vi "DivisionUI.vi"(0 "Divide in":refnum<class "Divide.lvclass">, 1 "B":dbl, 5 "A":dbl, 7 "user event out":refnum<user-event>, 9 "event source":refnum<user-event>, 11 "error in (no error)":errorcluster, 12 "Calculate":bool) -> (4 "Divide out":refnum<class "Divide.lvclass">, 6 "C":dbl, 15 "error out":errorcluster)   [LabVIEW 2023, in "Divide.lvclass"]
uses:
  Divide.lvclass
  C:/Users/santharu.subramanian/Documents/LV New Assignments/DVR in OOPS/Classes/Arithmetic/Arithmetic.lvclass
  Arithmetic/Arithmetic.lvclass
  Divide.lvclass/Divide.ctl
panel:
  # "DIVISION"
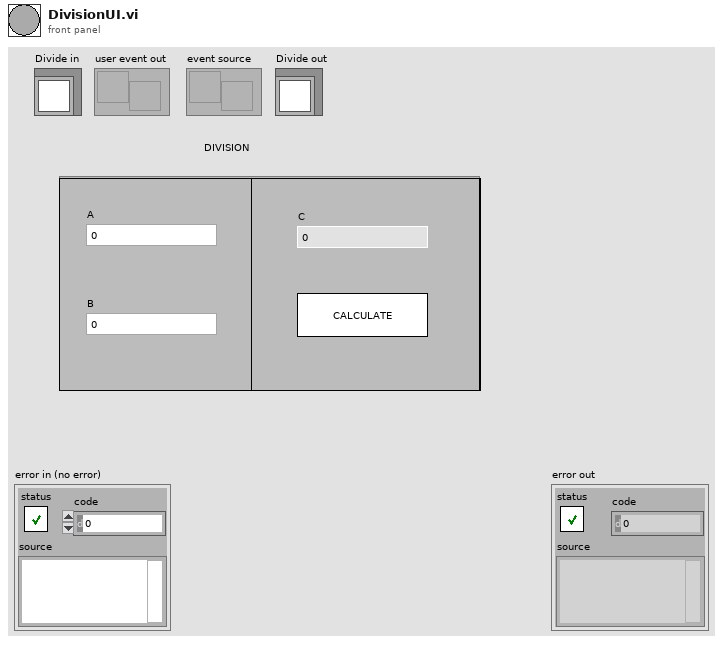
[diagram p1: front panel]
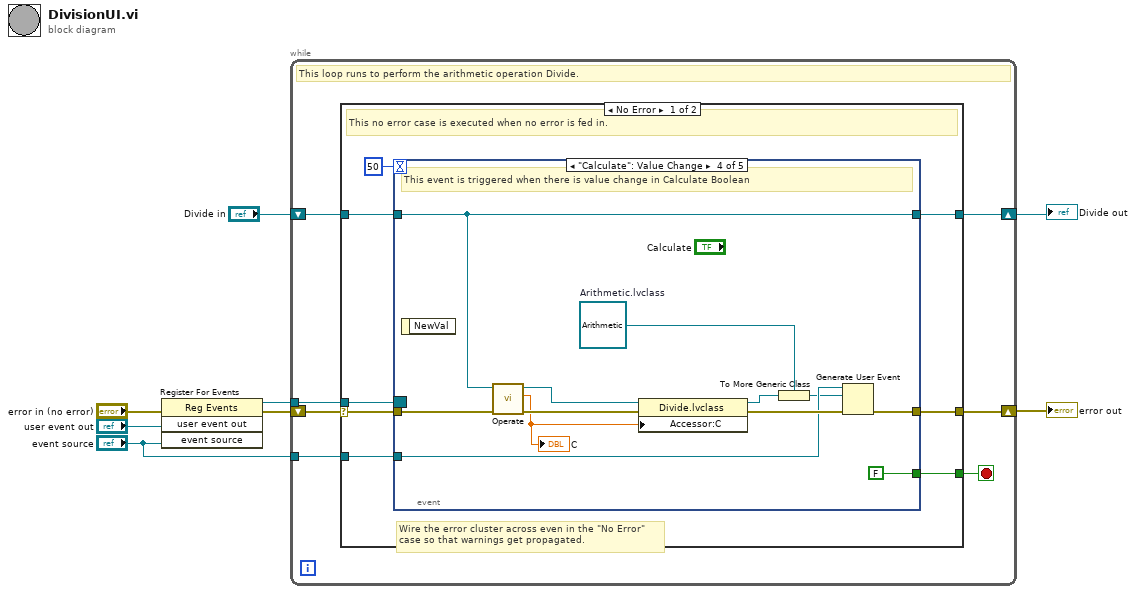
[diagram p0: block diagram]
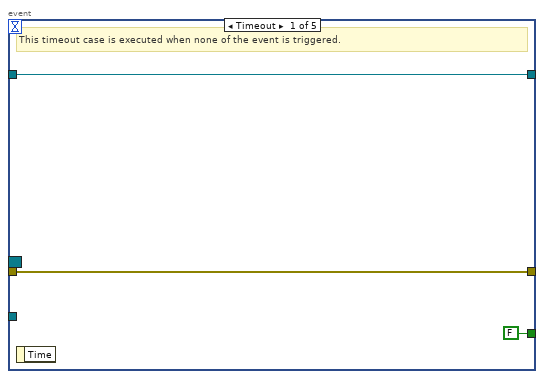
[diagram p2: hidden frame]
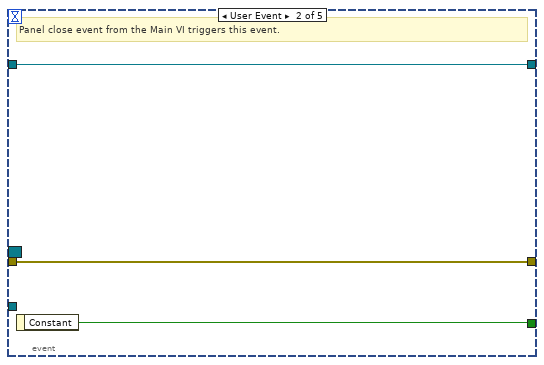
[diagram p3: hidden frame]
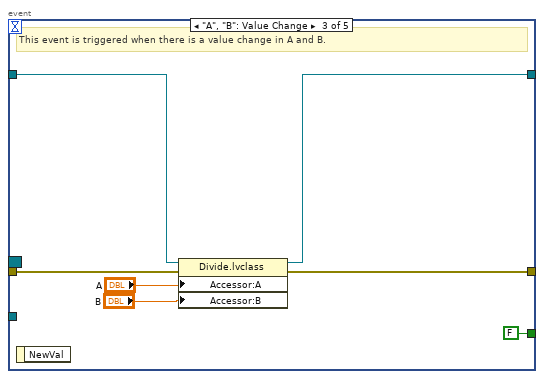
[diagram p4: hidden frame]
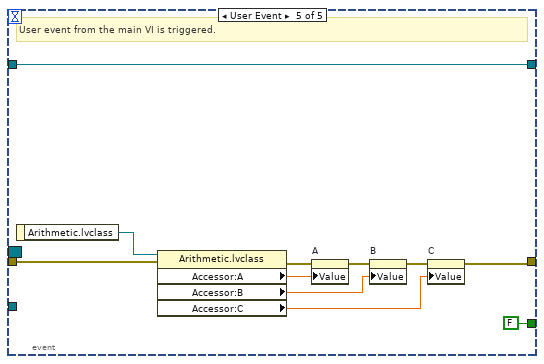
[diagram p5: hidden frame]
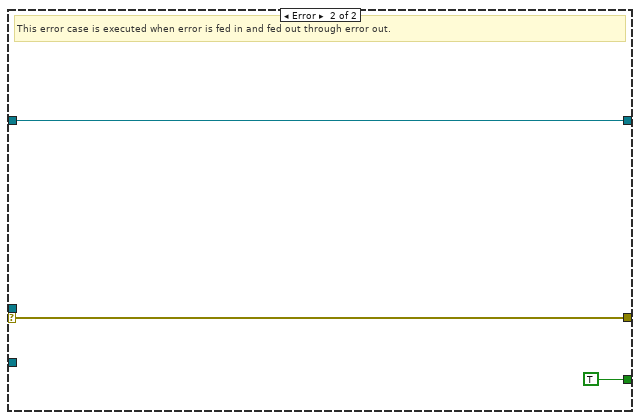
[diagram p6: hidden frame]
diagram:
  # "Wire the error cluster across even in the \"No Error\"\ncase so that warnings get propagated."
  n1 = register-events(error in="error in (no error)", "user event out", "event source") -> (reference out=w3:refnum<event-registration>, error out=w4:errorcluster)  [unwired: 1 in]
  n2 = while {
    shift-right: [w14] -> w6
    shift-left: w4 -> [w15]
    shift-right: [w12] -> w7
    shift-left: "Divide in" -> [w13]
    tunnel: w3 -> [w11]
    tunnel: "event source" -> [w9]
    stop <- w10 stop-if-true
    # "This loop runs to perform the arithmetic operation Divide."
    n3 = case shown="No Error" w15 {
      selector: w15 -> [w23 w62]
      tunnel: [w22 w62] -> w14
      tunnel: [w20 w61] -> w12
      tunnel: w13 -> [w21 w61]
      tunnel: w11 -> [w18 _]
      tunnel: [w17 TRUE] -> w10
      tunnel: w9 -> [w16 _]
      frame No Error {
        # "This no error case is executed when no error is fed in."
        n4 = event shown="[3] \"Calculate\": Value Change" {
          selector: w18 -> [_ _ _ _ _]
          dyn-events: _ -> [_ _ _ _ _]
          timeout: 50 -> [_ _ _ _ _]
          tunnel: w23 -> [w26 w29 w35 w48 w51]
          tunnel: [w26 w29 w34 w42 w50] -> w22
          tunnel: w21 -> [w25 w28 w36 w37 w59]
          tunnel: [w25 w28 w31 w37 w59] -> w20
          tunnel: [FALSE w27 FALSE FALSE FALSE ("Constant")] -> w17
          tunnel: w16 -> [_ _ _ w40 _]
          event Timeout {
            # "This timeout case is executed when none of the event is triggered."
            n5 = event-data() -> ()  [unwired: 1 in, 1 out]
          }
          event User Event {
            # "Panel close event from the Main VI triggers this event."
            n6 = event-data() -> ("Constant"=w27:bool)  [unwired: 1 in]
          }
          event "A", "B": Value Change {
            # "This event is triggered when there is a value change in A and B."
            n7 = event-data() -> ()  [unwired: 1 in, 1 out]
            n8 = property class="Divide.lvclass"(reference=w36, error in=w35, "Accessor:A"="A", "Accessor:B"="B") -> (reference out=w31:refnum<class "Divide.lvclass">, error out=w34:errorcluster)
          }
          event "Calculate": Value Change {
            w38 = refnum<class "Arithmetic.lvclass"> refnum  # Arithmetic.lvclass
            # "This event is triggered when there is value change in Calculate Boolean"
            n9 = event-data() -> ()  [unwired: 1 in, 1 out]
            n10 = call-dynamic "Operate.vi"("error in (no error)"=w48, "Divide in"=w37) -> ("error out"=w43:errorcluster, "C"=w41:dbl, "Divide out"=w44:refnum<class "Divide.lvclass">)  [unwired: 7 in]
            "C" <- w41
            n11 = property class="Divide.lvclass"(reference=w44, error in=w43, "Accessor:C"=w41) -> (reference out=w45:refnum<class "Divide.lvclass">, error out=w46:errorcluster)
            n12 = To More Generic Class(target class=w38, reference=w45) -> (generic class reference=w39:refnum<class "Arithmetic.lvclass">)
            n13 = Generate User Event(user event=w40, event data cluster=w39, error in=w46) -> (error out=w42:errorcluster)  [unwired: 1 in, 1 out]
          }
          event User Event {
            # "User event from the main VI is triggered."
            n14 = event-data() -> ("Arithmetic.lvclass"=w52:refnum<class "Arithmetic.lvclass">)  [unwired: 1 in]
            n15 = property class="Arithmetic.lvclass"(reference=w52, error in=w51) -> (error out=w58:errorcluster, "Accessor:A"=w57:dbl, "Accessor:B"=w54:dbl, "Accessor:C"=w53:dbl)  [unwired: 1 out]
            n16 = property on="A" class="DigNum (strict)"(error in=w58, "Value"=w57) -> (error out=w56:errorcluster)  [unwired: 1 in, 1 out]
            n17 = property on="B" class="DigNum (strict)"(error in=w56, "Value"=w54) -> (error out=w55:errorcluster)  [unwired: 1 in, 1 out]
            n18 = property on="C" class="DigNum (strict)"(error in=w55, "Value"=w53) -> (error out=w50:errorcluster)  [unwired: 1 in, 1 out]
          }
        }
      }
      frame Error {
        # "This error case is executed when error is fed in and fed out through error out."
      }
    }
  }
  "error out" <- w6
  "Divide out" <- w7
